vi "Graph_Water_Velocity(Subvi).vi"(2 "GPS_ItemNames":string[][](array[string]), 5 "Velocity_ItemNames":string[][](array[string])) -> (8 "1_2_Water_Velocity":dbl, 9 "1_2_Averange_SoundSpeed":dbl, 10 "1_3_Water_Velocity":dbl, 11 "1_3Averange_SoundSpeed":dbl, 12 "1_4_Water_Velocity":dbl, 13 "1_4_Averange_SoundSpeed":dbl, 14 "1_5_Water_Velocity":dbl, 15 "1_5_Averange_SoundSpeed":dbl, 16 "2_3_Water_Velocity":dbl, 17 "2_3_Averange_SoundSpeed":dbl, 18 "2_4_Water_Velocity":dbl, 19 "2_4_Averange_SoundSpeed":dbl, 20 "2_5_Water_Velocity":dbl, 21 "3_4_Water_Velocity":dbl, 22 "3_5_Water_Velocity":dbl, 23 "4_5_Water_Velocity":dbl, 24 "4_5_Averange_SoundSpeed":dbl, 25 "3_5_Averange_SoundSpeed":dbl, 26 "3_4_Averange_SoundSpeed":dbl, 27 "2_5_Averange_SoundSpeed":dbl)   [LabVIEW 2024]
panel:
  out "숫자 2":i32
  out "숫자":i32
  out "2_4_distance[m]":dbl
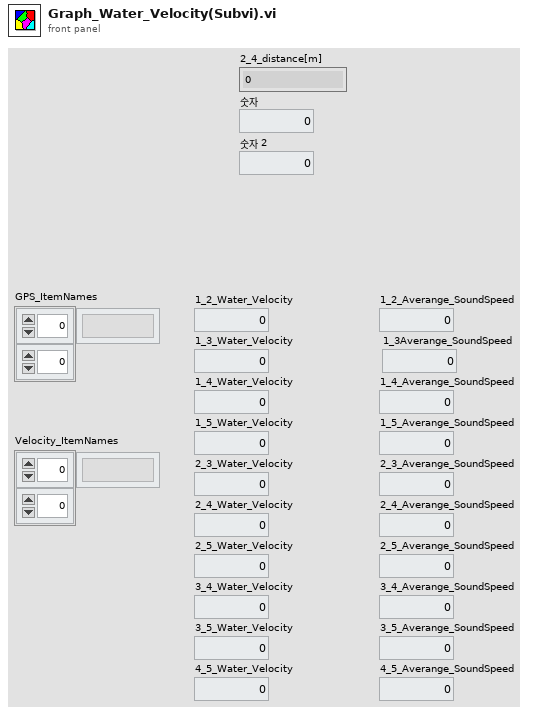
[diagram p1: front panel]
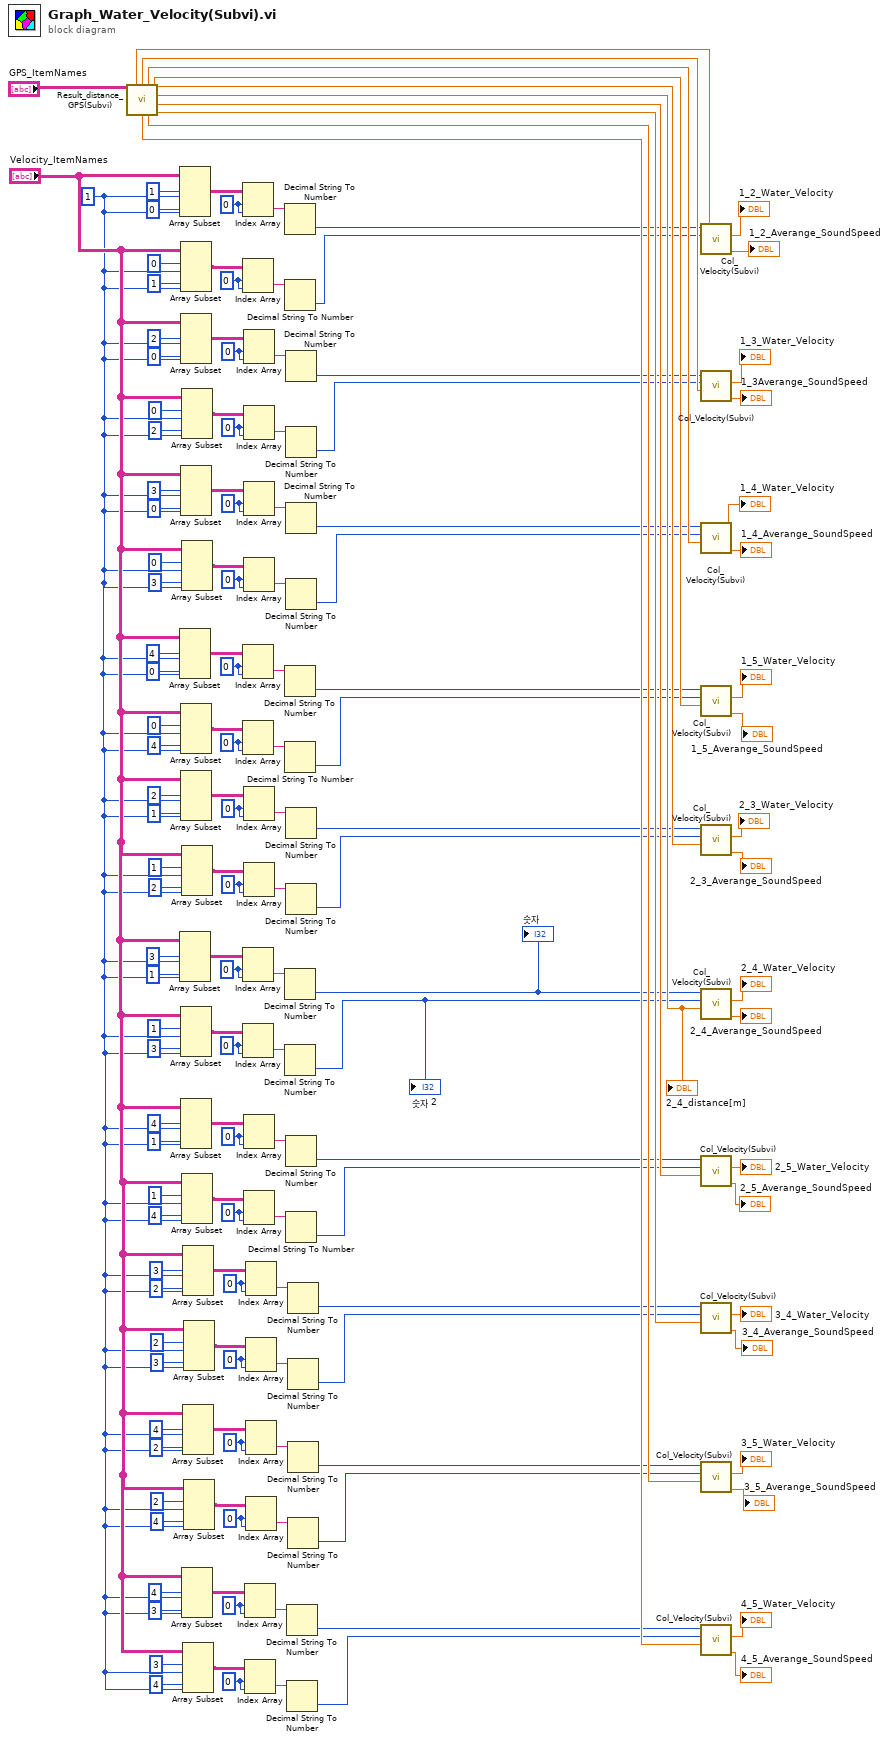
[diagram p0: block diagram]
diagram:
  w130 = 0 ("인덱스 (행)")
  w133 = 0 ("인덱스 (행)")
  w124 = 0 ("인덱스 (행)")
  w121 = 0 ("인덱스 (행)")
  w104 = 0 ("인덱스 (행)")
  w107 = 0 ("인덱스 (행)")
  w98 = 0 ("인덱스 (행)")
  w95 = 0 ("인덱스 (행)")
  w78 = 0 ("인덱스 (행)")
  w81 = 0 ("인덱스 (행)")
  w72 = 0 ("인덱스 (행)")
  w69 = 0 ("인덱스 (행)")
  w52 = 0 ("인덱스 (행)")
  w55 = 0 ("인덱스 (행)")
  w46 = 0 ("인덱스 (행)")
  w43 = 0 ("인덱스 (행)")
  w26 = 0 ("인덱스 (행)")
  w29 = 0 ("인덱스 (행)")
  w20 = 0 ("인덱스 (행)")
  w17 = 0 ("인덱스 (행)")
  w139 = 1 ("길이")
  n1 = call "Result_distance_GPS(Subvi).vi"("아이템 이름"="GPS_ItemNames") -> ("1_2_distance[m]"=w24:dbl, "1_3_distance[m]"=w37:dbl, "1_4_distance[m]"=w50:dbl, "1_5_distance[m]"=w63:dbl, "2_3_distance[m]"=w76:dbl, "2_4_distance[m]"=w89:dbl, "2_5_distance[m]"=w102:dbl, "4_5_distance[m]"=w142:dbl, "3_5_distance[m]"=w128:dbl, "3_4_distance[m]"=w115:dbl)  [unwired: 5 in]
  "2_4_distance[m]" <- w89
  n2 = Array Subset(array="Velocity_ItemNames", index (row)=1 ("인덱스"), length (row)=w139, index (col)=0 ("인덱스"), length (col)=w139) -> (w16:string[][])
  n3 = Array Subset(array="Velocity_ItemNames", index (row)=4 ("인덱스"), length (row)=w139, index (col)=0 ("인덱스"), length (col)=w139) -> (w56:string[][])
  n4 = Array Subset(array="Velocity_ItemNames", index (row)=3 ("인덱스"), length (row)=w139, index (col)=1 ("인덱스"), length (col)=w139) -> (w82:string[][])
  n5 = Array Subset(array="Velocity_ItemNames", index (row)=0 ("인덱스"), length (row)=w139, index (col)=1 ("인덱스"), length (col)=w139) -> (w21:string[][])
  n6 = Array Subset(array="Velocity_ItemNames", index (row)=2 ("인덱스"), length (row)=w139, index (col)=0 ("인덱스"), length (col)=w139) -> (w30:string[][])
  n7 = Array Subset(array="Velocity_ItemNames", index (row)=3 ("인덱스"), length (row)=w139, index (col)=0 ("인덱스"), length (col)=w139) -> (w42:string[][])
  n8 = Array Subset(array="Velocity_ItemNames", index (row)=0 ("인덱스"), length (row)=w139, index (col)=4 ("인덱스"), length (col)=w139) -> (w51:string[][])
  n9 = Array Subset(array="Velocity_ItemNames", index (row)=2 ("인덱스"), length (row)=w139, index (col)=1 ("인덱스"), length (col)=w139) -> (w68:string[][])
  n10 = Array Subset(array="Velocity_ItemNames", index (row)=1 ("인덱스"), length (row)=w139, index (col)=3 ("인덱스"), length (col)=w139) -> (w77:string[][])
  n11 = Array Subset(array="Velocity_ItemNames", index (row)=4 ("인덱스"), length (row)=w139, index (col)=1 ("인덱스"), length (col)=w139) -> (w94:string[][])
  n12 = Array Subset(array="Velocity_ItemNames", index (row)=0 ("인덱스"), length (row)=w139, index (col)=2 ("인덱스"), length (col)=w139) -> (w25:string[][])
  n13 = Array Subset(array="Velocity_ItemNames", index (row)=0 ("인덱스"), length (row)=w139, index (col)=3 ("인덱스"), length (col)=w139) -> (w47:string[][])
  n14 = Array Subset(array="Velocity_ItemNames", index (row)=1 ("인덱스"), length (row)=w139, index (col)=2 ("인덱스"), length (col)=w139) -> (w73:string[][])
  n15 = Array Subset(array="Velocity_ItemNames", index (row)=1 ("인덱스"), length (row)=w139, index (col)=4 ("인덱스"), length (col)=w139) -> (w99:string[][])
  n16 = Array Subset(array="Velocity_ItemNames", index (row)=4 ("인덱스"), length (row)=w139, index (col)=3 ("인덱스"), length (col)=w139) -> (w134:string[][])
  n17 = Array Subset(array="Velocity_ItemNames", index (row)=3 ("인덱스"), length (row)=w139, index (col)=2 ("인덱스"), length (col)=w139) -> (w108:string[][])
  n18 = Array Subset(array="Velocity_ItemNames", index (row)=4 ("인덱스"), length (row)=w139, index (col)=2 ("인덱스"), length (col)=w139) -> (w120:string[][])
  n19 = Array Subset(array="Velocity_ItemNames", index (row)=3 ("인덱스"), length (row)=w139, index (col)=4 ("인덱스"), length (col)=w139) -> (w129:string[][])
  n20 = Array Subset(array="Velocity_ItemNames", index (row)=2 ("인덱스"), length (row)=w139, index (col)=3 ("인덱스"), length (col)=w139) -> (w103:string[][])
  n21 = Array Subset(array="Velocity_ItemNames", index (row)=2 ("인덱스"), length (row)=w139, index (col)=4 ("인덱스"), length (col)=w139) -> (w125:string[][])
  n22 = Index Array(array=w16, index (row)=w17, index (col)=w17) -> (element=w18:string)
  n23 = Index Array(array=w21, index (row)=w20, index (col)=w20) -> (element=w19:string)
  n24 = Index Array(array=w56, index (row)=w55, index (col)=w55) -> (element=w54:string)
  n25 = Index Array(array=w51, index (row)=w52, index (col)=w52) -> (element=w53:string)
  n26 = Index Array(array=w82, index (row)=w81, index (col)=w81) -> (element=w80:string)
  n27 = Index Array(array=w77, index (row)=w78, index (col)=w78) -> (element=w79:string)
  n28 = Index Array(array=w30, index (row)=w29, index (col)=w29) -> (element=w28:string)
  n29 = Index Array(array=w25, index (row)=w26, index (col)=w26) -> (element=w27:string)
  n30 = Index Array(array=w42, index (row)=w43, index (col)=w43) -> (element=w44:string)
  n31 = Index Array(array=w47, index (row)=w46, index (col)=w46) -> (element=w45:string)
  n32 = Index Array(array=w68, index (row)=w69, index (col)=w69) -> (element=w70:string)
  n33 = Index Array(array=w73, index (row)=w72, index (col)=w72) -> (element=w71:string)
  n34 = Index Array(array=w94, index (row)=w95, index (col)=w95) -> (element=w96:string)
  n35 = Index Array(array=w99, index (row)=w98, index (col)=w98) -> (element=w97:string)
  n36 = Index Array(array=w134, index (row)=w133, index (col)=w133) -> (element=w132:string)
  n37 = Index Array(array=w129, index (row)=w130, index (col)=w130) -> (element=w131:string)
  n38 = Index Array(array=w108, index (row)=w107, index (col)=w107) -> (element=w106:string)
  n39 = Index Array(array=w103, index (row)=w104, index (col)=w104) -> (element=w105:string)
  n40 = Index Array(array=w120, index (row)=w121, index (col)=w121) -> (element=w122:string)
  n41 = Index Array(array=w125, index (row)=w124, index (col)=w124) -> (element=w123:string)
  n42 = Decimal String To Number(string=w18) -> (number=w22:i32)  [unwired: 2 in, 1 out]
  n43 = Decimal String To Number(string=w19) -> (number=w23:i32)  [unwired: 2 in, 1 out]
  n44 = Decimal String To Number(string=w54) -> (number=w61:i32)  [unwired: 2 in, 1 out]
  n45 = Decimal String To Number(string=w53) -> (number=w62:i32)  [unwired: 2 in, 1 out]
  n46 = Decimal String To Number(string=w80) -> (number=w87:i32)  [unwired: 2 in, 1 out]
  "숫자" <- w87
  n47 = Decimal String To Number(string=w79) -> (number=w88:i32)  [unwired: 2 in, 1 out]
  "숫자 2" <- w88
  n48 = Decimal String To Number(string=w28) -> (number=w35:i32)  [unwired: 2 in, 1 out]
  n49 = Decimal String To Number(string=w27) -> (number=w36:i32)  [unwired: 2 in, 1 out]
  n50 = Decimal String To Number(string=w44) -> (number=w48:i32)  [unwired: 2 in, 1 out]
  n51 = Decimal String To Number(string=w45) -> (number=w49:i32)  [unwired: 2 in, 1 out]
  n52 = Decimal String To Number(string=w70) -> (number=w74:i32)  [unwired: 2 in, 1 out]
  n53 = Decimal String To Number(string=w71) -> (number=w75:i32)  [unwired: 2 in, 1 out]
  n54 = Decimal String To Number(string=w96) -> (number=w100:i32)  [unwired: 2 in, 1 out]
  n55 = Decimal String To Number(string=w97) -> (number=w101:i32)  [unwired: 2 in, 1 out]
  n56 = Decimal String To Number(string=w132) -> (number=w140:i32)  [unwired: 2 in, 1 out]
  n57 = Decimal String To Number(string=w131) -> (number=w141:i32)  [unwired: 2 in, 1 out]
  n58 = Decimal String To Number(string=w106) -> (number=w113:i32)  [unwired: 2 in, 1 out]
  n59 = Decimal String To Number(string=w105) -> (number=w114:i32)  [unwired: 2 in, 1 out]
  n60 = Decimal String To Number(string=w122) -> (number=w126:i32)  [unwired: 2 in, 1 out]
  n61 = Decimal String To Number(string=w123) -> (number=w127:i32)  [unwired: 2 in, 1 out]
  n62 = call "Col_Velocity(Subvi).vi"("거리"=w24, "Station_index_2"=w23, "Station_index_1"=w22) -> ("Averange_SoundSpeed"=→"1_2_Averange_SoundSpeed":dbl, "Water_Velocity"=→"1_2_Water_Velocity":dbl)  [unwired: 7 in]
  n63 = call "Col_Velocity(Subvi).vi"("거리"=w37, "Station_index_2"=w36, "Station_index_1"=w35) -> ("Averange_SoundSpeed"=→"1_3Averange_SoundSpeed":dbl, "Water_Velocity"=→"1_3_Water_Velocity":dbl)  [unwired: 7 in]
  n64 = call "Col_Velocity(Subvi).vi"("거리"=w50, "Station_index_2"=w49, "Station_index_1"=w48) -> ("Averange_SoundSpeed"=→"1_4_Averange_SoundSpeed":dbl, "Water_Velocity"=→"1_4_Water_Velocity":dbl)  [unwired: 7 in]
  n65 = call "Col_Velocity(Subvi).vi"("거리"=w63, "Station_index_2"=w62, "Station_index_1"=w61) -> ("Averange_SoundSpeed"=→"1_5_Averange_SoundSpeed":dbl, "Water_Velocity"=→"1_5_Water_Velocity":dbl)  [unwired: 7 in]
  n66 = call "Col_Velocity(Subvi).vi"("거리"=w76, "Station_index_2"=w75, "Station_index_1"=w74) -> ("Averange_SoundSpeed"=→"2_3_Averange_SoundSpeed":dbl, "Water_Velocity"=→"2_3_Water_Velocity":dbl)  [unwired: 7 in]
  n67 = call "Col_Velocity(Subvi).vi"("거리"=w89, "Station_index_2"=w88, "Station_index_1"=w87) -> ("Averange_SoundSpeed"=→"2_4_Averange_SoundSpeed":dbl, "Water_Velocity"=→"2_4_Water_Velocity":dbl)  [unwired: 7 in]
  n68 = call "Col_Velocity(Subvi).vi"("거리"=w102, "Station_index_2"=w101, "Station_index_1"=w100) -> ("Averange_SoundSpeed"=→"2_5_Averange_SoundSpeed":dbl, "Water_Velocity"=→"2_5_Water_Velocity":dbl)  [unwired: 7 in]
  n69 = call "Col_Velocity(Subvi).vi"("거리"=w115, "Station_index_2"=w114, "Station_index_1"=w113) -> ("Averange_SoundSpeed"=→"3_4_Averange_SoundSpeed":dbl, "Water_Velocity"=→"3_4_Water_Velocity":dbl)  [unwired: 7 in]
  n70 = call "Col_Velocity(Subvi).vi"("거리"=w128, "Station_index_2"=w127, "Station_index_1"=w126) -> ("Averange_SoundSpeed"=→"3_5_Averange_SoundSpeed":dbl, "Water_Velocity"=→"3_5_Water_Velocity":dbl)  [unwired: 7 in]
  n71 = call "Col_Velocity(Subvi).vi"("거리"=w142, "Station_index_2"=w141, "Station_index_1"=w140) -> ("Averange_SoundSpeed"=→"4_5_Averange_SoundSpeed":dbl, "Water_Velocity"=→"4_5_Water_Velocity":dbl)  [unwired: 7 in]
